vi "open connection.vi"(6 "timeout ms (60000)":i32, 8 "error in (no error)":errorcluster, 9 "service name":string, 10 "port":u16, 11 "address":string) -> (0 "error out":errorcluster, 3 "TCP Network Connection out":refnum<k5>)   [LabVIEW 2015, in "TCP client.lvclass"]
uses:
  TCP client.lvclass
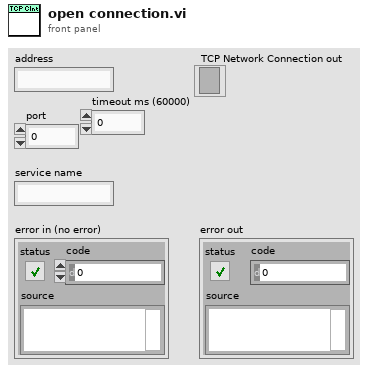
[diagram p1: front panel]
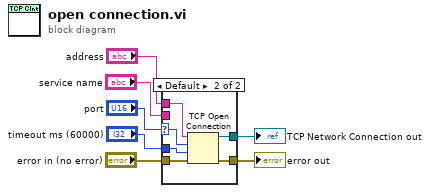
[diagram p0: block diagram]
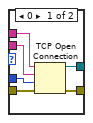
[diagram p2: hidden frame]
diagram:
  n1 = case shown="Default" "port" {
    selector: "port" -> [_ w16]
    tunnel: "address" -> [w13 w19]
    tunnel: "service name" -> [w12 _]
    tunnel: [w11 w17] -> w7
    tunnel: [w10 w18] -> w6
    tunnel: "error in (no error)" -> [w8 w15]
    tunnel: "timeout ms (60000)" -> [w9 w14]
    frame 0 {
      n2 = TCP Open Connection(address=w13, remote port or service name=w12, timeout ms (60000)=w9, error in (no error)=w8) -> (connection ID=w10:refnum<k5>, error out=w11:errorcluster)  [unwired: 1 in]
    }
    frame Default {
      n3 = TCP Open Connection(address=w19, remote port or service name=w16, timeout ms (60000)=w14, error in (no error)=w15) -> (connection ID=w18:refnum<k5>, error out=w17:errorcluster)  [unwired: 1 in]
    }
  }
  "error out" <- w7
  "TCP Network Connection out" <- w6
